vi "createMsgBuilder.vi"(8 "error in (no error)":errorcluster, 11 "path in":path=path "C:/dev/Hexagon-VTD-Custom-Device/Libraries/VC.dll") -> (0 "error out":errorcluster, 3 "builderHandle":u64)   [LabVIEW 2023, in "RDB.lvlib"]
uses:
  RDB.lvlib
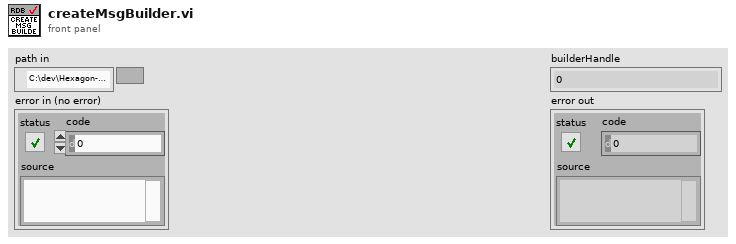
[diagram p1: front panel]
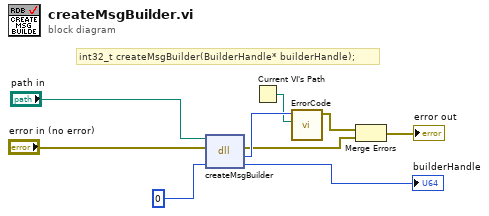
[diagram p0: block diagram]
diagram:
  # "int32_t createMsgBuilder(BuilderHandle* builderHandle);"
  n1 = dll-call lib="C:/dev/Hexagon-VTD-Custom-Device/Libraries/libVC.dll" fn="createMsgBuilder"(path in="path in", error in="error in (no error)", "builderHandle"=u64 0) -> (error out=w3:errorcluster, "return type"=w5:i32, "builderHandle"=→"builderHandle":u64)  [unwired: 1 in, 1 out]
  n2 = Current VI's Path() -> (path=w1:path)
  n3 = call "ErrorCode.vi"("parent VI path"=w1, "return type"=w5) -> ("error out"=w4:errorcluster)  [unwired: 9 in]
  n4 = Merge Errors(w4, w3) -> (→"error out":errorcluster)
